vi "mount share.vi"(8 "Error In":errorcluster, 9 "share":string="UserMagnetData", 10 "Server":string="bandicoot", 11 "Mount point":string="Y:") -> (0 "Error Out":errorcluster, 3 "standard output":string)   [LabVIEW 2015]
panel:
  out "standard error":string
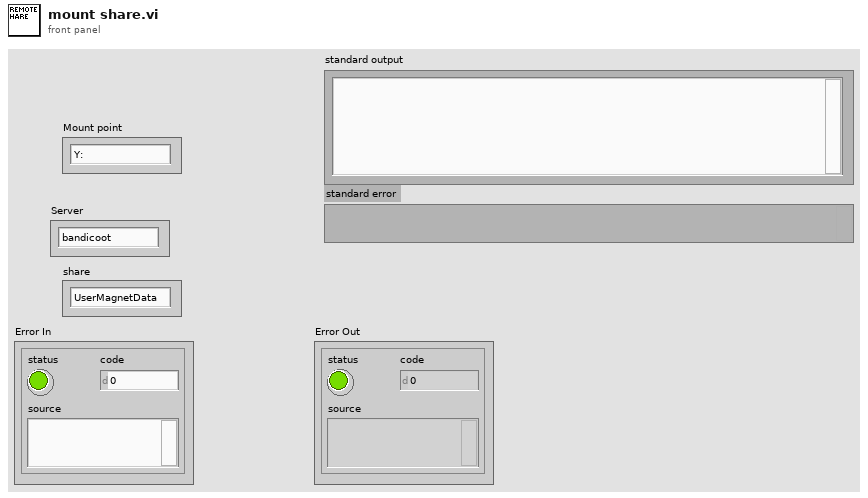
[diagram p1: front panel]
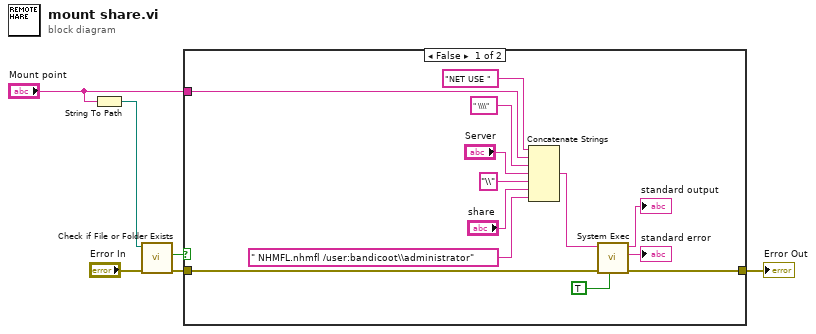
[diagram p0: block diagram]
diagram:
  n1 = String To Path(string="Mount point") -> (path=w4:path)
  n2 = call <vilib>:"Check if File or Folder Exists.vi"("error in (no error)"="Error In", "path"=w4) -> ("error out"=w2:errorcluster, "file or folder exists?"=w1:bool)  [unwired: 7 in, 1 out]
  n3 = case shown="False" w1 {
    tunnel: [w7 w20] -> w6
    tunnel: "Mount point" -> [w9 _]
    tunnel: w2 -> [w8 w20]
    frame False {
      n4 = Concatenate Strings("NET USE " ("string"), w9, " \\\\" ("string"), "Server", "\\" ("string"), "share", " NHMFL.nhmfl /user:bandicoot\\administrator" ("string")) -> (w17:string)
      n5 = call <vilib>:"System Exec.vi"("run minimized? (F)"=TRUE, "error in (no error)"=w8, "command line"=w17) -> ("error out"=w7:errorcluster, "standard error"=→"standard error":string, "standard output"=→"standard output":string)  [unwired: 5 in, 1 out]
    }
    frame True {
    }
  }
  "Error Out" <- w6
